vi "Set Config.vi"(7 "Column Type":T1, 8 "error in (no error)":errorcluster, 9 "Column Name":string, 10 "Table Name":string, 11 "Basic Column Configuration in":refnum<class "Basic Column Configuration.lvclass">) -> (0 "error out":errorcluster, 3 "Basic Column Configuration out":refnum<class "Basic Column Configuration.lvclass">)   [LabVIEW 2020, in "Basic Columns.lvlib" / "Basic Column Configuration.lvclass"]
uses:
  Basic Column Configuration.lvclass
  Database Interfaces/Database data type.ctl
  Basic Column Configuration.lvclass/Basic Column Configuration.ctl
  Database Interfaces.lvlib
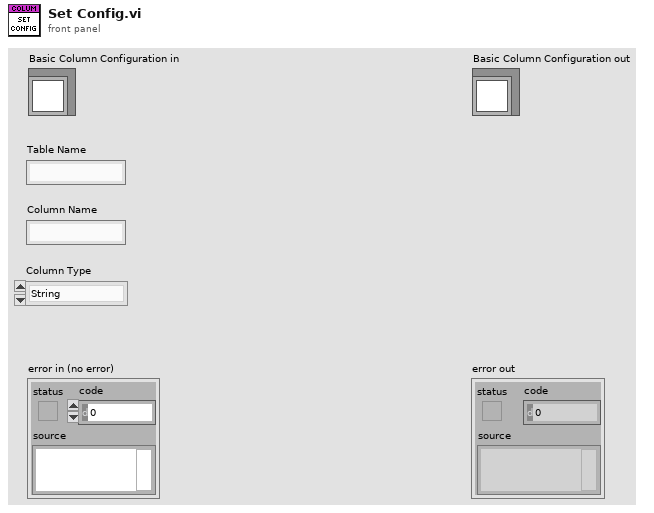
[diagram p1: front panel]
types:
  T1 = typedef "Database Interfaces.lvlib/Database data type.ctl" = enum16{"String", "Long (I32)", "Single (SGL)", "Double (DBL)", "Date/Time", "Binary"}
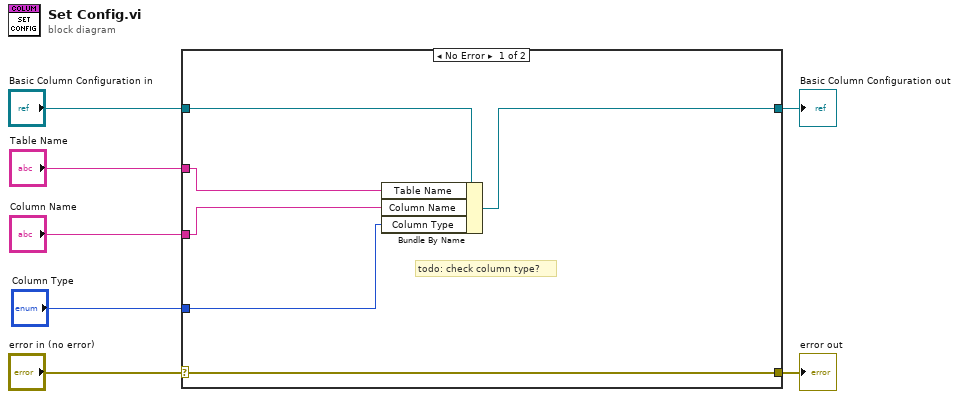
[diagram p0: block diagram]
diagram:
  n1 = case shown="No Error" "error in (no error)" {
    selector: "error in (no error)" -> [w13 w15]
    tunnel: [w13 w15] -> w6
    tunnel: [w11 w14] -> w4
    tunnel: "Basic Column Configuration in" -> [w12 w14]
    tunnel: "Table Name" -> [w10 _]
    tunnel: "Column Name" -> [w9 _]
    tunnel: "Column Type" -> [w8 _]
    frame No Error {
      # "todo: check column type?"
      n2 = Bundle By Name(cluster=w12, "Table Name"=w10, "Column Name"=w9, "Column Type"=w8) -> (w11:refnum<class "Basic Column Configuration.lvclass">)
    }
    frame Error {
    }
  }
  "error out" <- w6
  "Basic Column Configuration out" <- w4
